vi "set_interval.vi"(8 "error in (no error)":errorcluster, 10 "interval (1000 ms)":u32=1000, 11 "timer in":refnum<class "rytimer.lvclass">) -> (0 "error out":errorcluster, 3 "timer out":refnum<class "rytimer.lvclass">)   [LabVIEW 2017, in "rytimer.lvclass"]
uses:
  rytimer.lvclass
  rytimer.lvclass/rytimer.ctl
  state.ctl
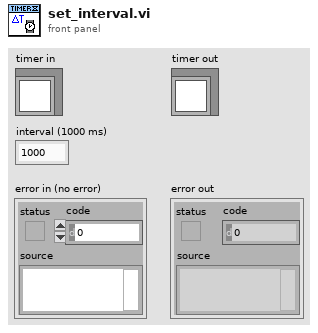
[diagram p1: front panel]
types:
  T1 = typedef "rytimer.lvclass/state.ctl" = enum8{"stop", "start", "mode", "interval", "message"}
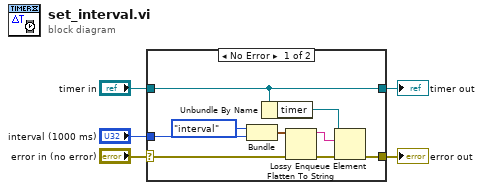
[diagram p0: block diagram]
diagram:
  n1 = case shown="No Error" "error in (no error)" {
    selector: "error in (no error)" -> [w13 w16]
    tunnel: "interval (1000 ms)" -> [w14 _]
    tunnel: [w12 w16] -> w3
    tunnel: "timer in" -> [w6 w15]
    tunnel: [w6 w15] -> w1
    frame No Error {
      n2 = Bundle("state"=state."interval", "interval (1000 ms)"=w14) -> (w8:cluster{"state":T1, "interval (1000 ms)":u32})  [unwired: 1 in]
      n3 = Unbundle By Name(w6) -> ("timer"=w7:refnum<queue>)
      n4 = Flatten To String(anything=w8, error in (no error)=w13) -> (data string=w9:string, error out=w10:errorcluster)  [unwired: 2 in, 1 out]
      n5 = Lossy Enqueue Element(queue=w7, element=w9, error in (no error)=w10) -> (error out=w12:errorcluster)  [unwired: 3 out]
    }
    frame Error {
    }
  }
  "error out" <- w3
  "timer out" <- w1
